vi "AStop_GO_test.vi"() -> ()   [LabVIEW 2011]
uses:
  <vilib>/Instr/_visa.llb/VISA Configure Serial Port (Instr).vi
panel:
  out "Error 13":errorcluster
  out "Error 28":errorcluster
  out "Error 25":errorcluster
  in  "delay (ms)":u32=333
  out "Epoque":dbl format="%.2f"
  in  "stop":bool
  out "DST?":bool
  out "error out":errorcluster
  in  "VISA resource name":refnum<visa-resource-name>="COM4"
  in  "baud rate (9600)":u32=57600
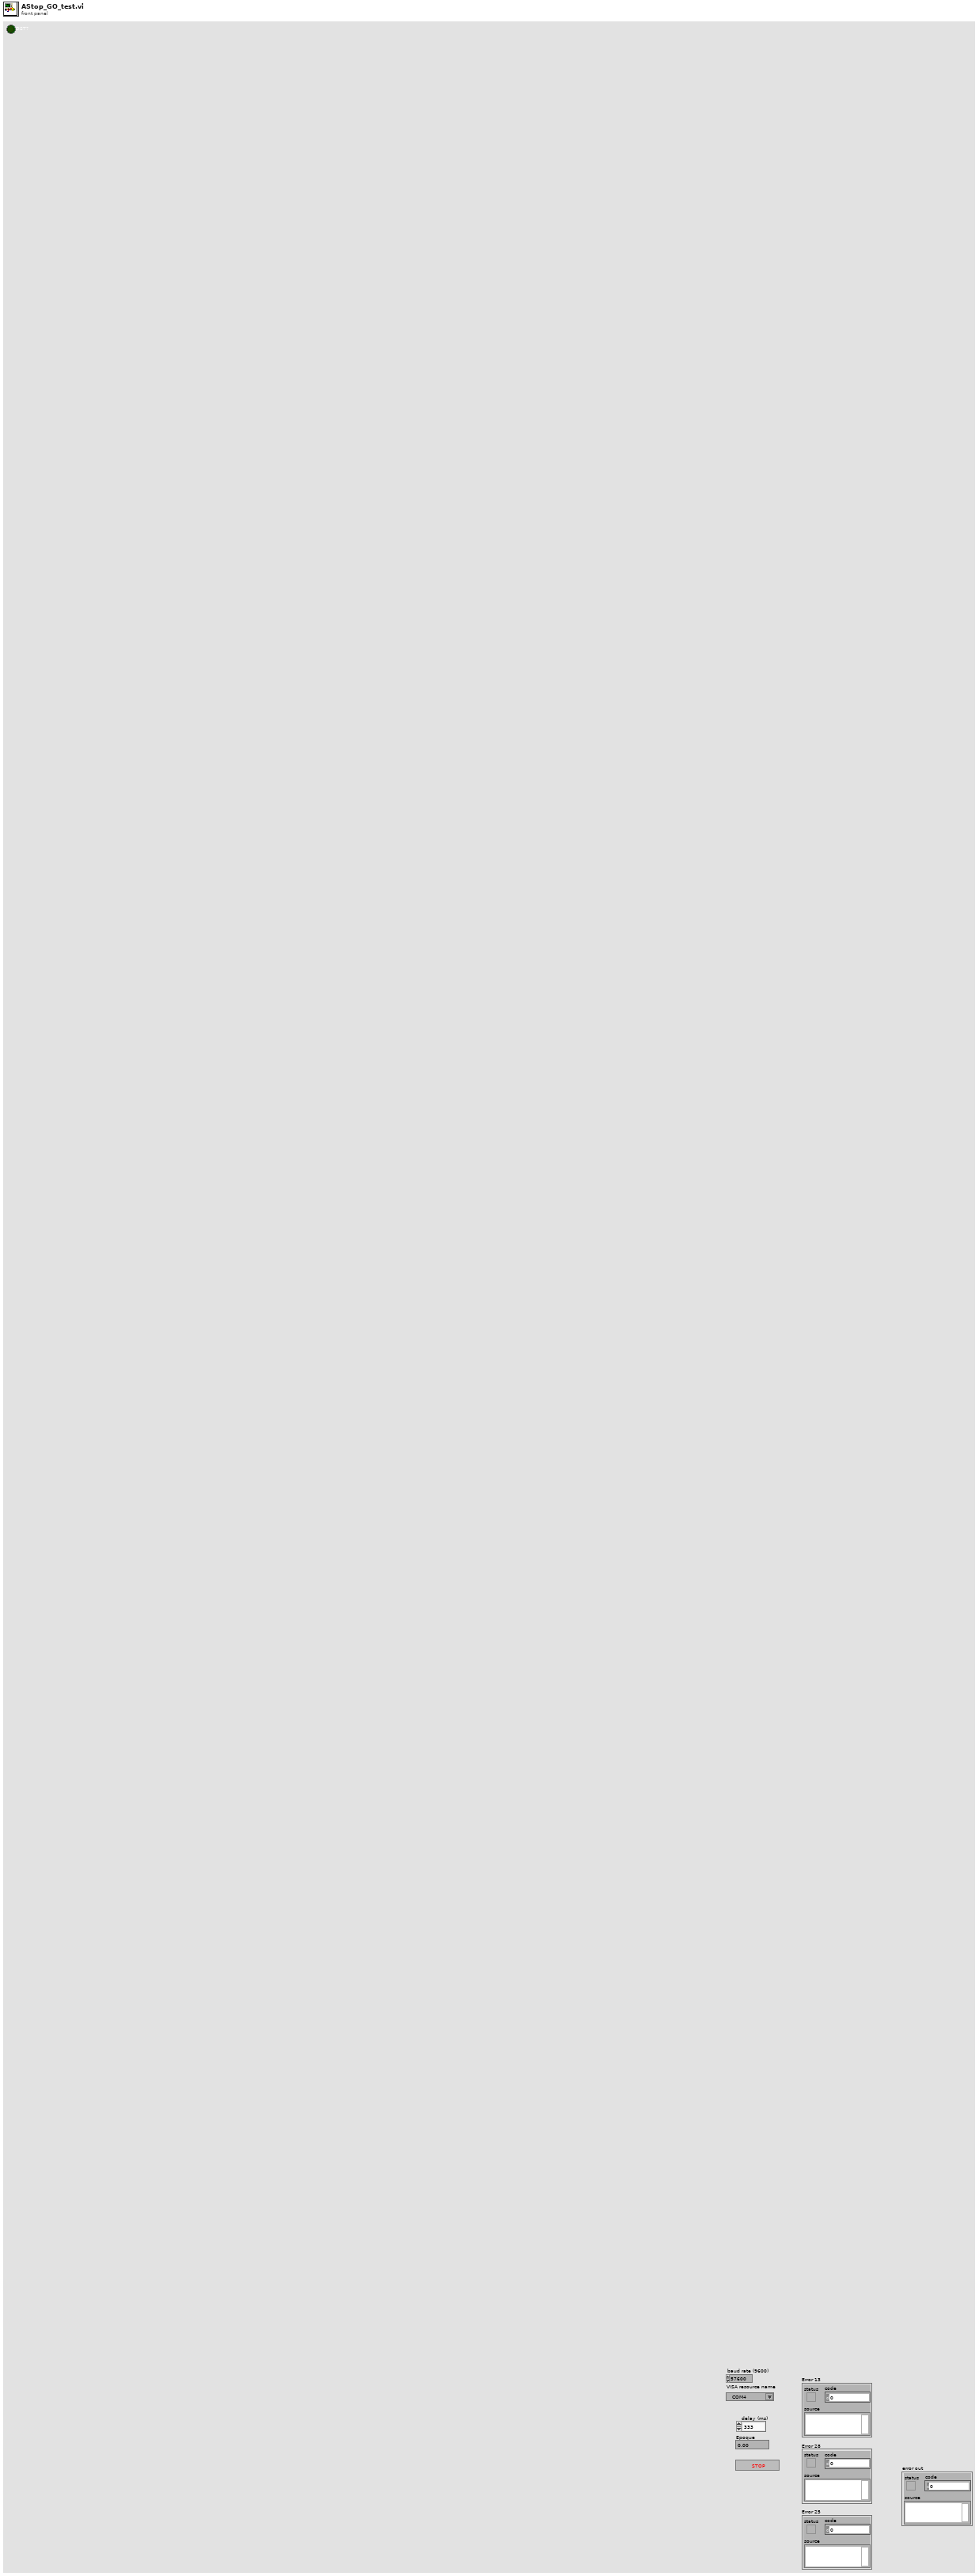
[diagram p1: front panel]
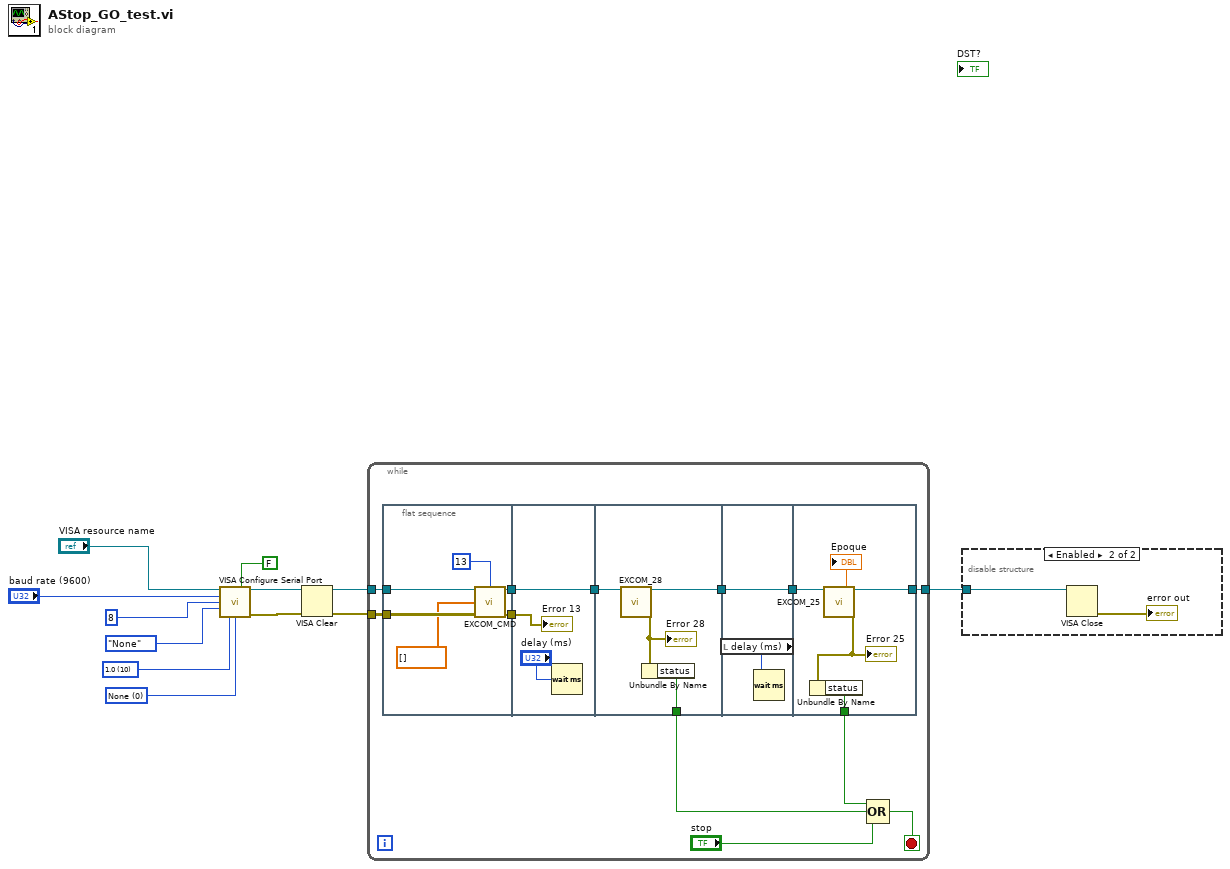
[diagram p0: block diagram]
diagram:
  w11 = u16 0 items=["None", "XON/XOFF", "RTS/CTS", "XON/XOFF & RTS/CTS", "DTR/DSR", "XON/XOFF & DTR/DSR"] ("flow control (0:none)")
  w10 = u16 10 items=["1.0"=10, "1.5"=15, "2.0"=20] ("stop bits (10: 1 bit)")
  n1 = call-poly "VISA Configure Serial Port"("VISA resource name"="VISA resource name", "Enable Termination\nChar (T)"=FALSE ("Enable Termination\nChar (T)"), "baud rate (9600)"="baud rate (9600)", "data bits (8)"=u16 8, "parity (0:none)"=enum16{"None", "Odd", "Even", "Mark", "Space"}."None", "stop bits (10: 1 bit)"=w10, "flow control (0:none)"=w11) -> ("VISA resource name out"=w5:refnum<visa-resource-name>, "error out"=w4:errorcluster)  [unwired: 7 in]
  n2 = VISA Clear(VISA resource name=w5, error in (no error)=w4) -> (VISA resource name out=w3:refnum<visa-resource-name>, error out=w2:errorcluster)
  n3 = while {
    tunnel: w3 -> [w24]
    tunnel: w2 -> [w23]
    tunnel: [w13] -> w1
    stop <- w22 stop-if-true
    n4 = flat-sequence {
      tunnel: w24 -> [w30]
      tunnel: w23 -> [w29]
      tunnel: [w26] -> w20
      tunnel: [w25] -> w19
      tunnel: w20 -> [w33]
      tunnel: w19 -> [w31]
      tunnel: [w33] -> w18
      tunnel: w18 -> [w37]
      tunnel: [w36] -> w17
      tunnel: [w35] -> w15
      tunnel: w17 -> [w39]
      tunnel: [w39] -> w16
      tunnel: w16 -> [w42]
      tunnel: [w43] -> w14
      tunnel: [w41] -> w13
      frame #0 {
        n5 = call "EXCOM_CMD.vi"("VRN IN"=w30, "Commande #"=13, "Args"=dbl[] [], "Error IN"=w29) -> ("VRN OUT"=w26:refnum<visa-resource-name>, "Error OUT"=w25:errorcluster)  [unwired: 9 in, 1 out]
      }
      frame #1 {
        n6 = Wait (ms)(milliseconds to wait="delay (ms)") -> ()  [unwired: 1 out]
        "Error 13" <- w31
      }
      frame #2 {
        n7 = call "EXCOM_28.vi"("VISA resource name"=w37) -> ("VISA resource name dup"=w36:refnum<visa-resource-name>, "Error OUT"=w34:errorcluster)  [unwired: 13 in, 4 out]
        "Error 28" <- w34
        n8 = Unbundle By Name(w34) -> ("status"=w35:bool)
      }
      frame #3 {
        n9 = local read "delay (ms)"() -> (w38:u32)
        n10 = Wait (ms)(milliseconds to wait=w38) -> ()  [unwired: 1 out]
      }
      frame #4 {
        n11 = call "EXCOM_25.vi"("VISA resource name"=w42) -> ("Epoque"=→"Epoque":dbl, "VISA resource name dup"=w41:refnum<visa-resource-name>, "Error OUT"=w40:errorcluster)  [unwired: 4 in, 12 out]
        "Error 25" <- w40
        n12 = Unbundle By Name(w40) -> ("status"=w43:bool)
      }
    }
    n13 = Compound Arithmetic op=OR(w14, w15, "stop") -> (w22:bool)
  }
  n14 = disable-structure shown="Enabled" {
    disable-tunnel: w1 -> [_ w46]
    frame Disabled {
    }
    frame Enabled {
      n15 = VISA Close(VISA resource name=w46) -> (error out=→"error out":errorcluster)  [unwired: 1 in]
    }
  }
